vi "Evaluate Sum of Exponentials.vi"(8 "error in (no error)":errorcluster, 10 "Ramp":dbl[](array[numeric]), 11 "Exp Parameters Array":T1[](array[typedef])) -> (0 "error out":errorcluster, 3 "Plot":T2)   [LabVIEW 2021, in "Fits.lvlib"]
doc: "Evaluates a sum of T-periodic exponential terms whose parameters are provided as an array of components (<B>Exp Parameters Array</B>).\n\nThe <B>baseline</B> parameter needs to be provided with the first component. Additional baseline parameters are ignored.\n\nThis VI computes the exponential term as exp(-(t - t_0)[T}/tau) if parameter <B>sigma</B> is NaN.\n\nOtherwise, the exponential term is computed as exp(-(t - t_0)[T]/sigma^2).\n\nThe sum is evaluated at locations provided in the <B>Ramp</B> array."
uses:
  Fits.lvlib
  Graphs/XY Graph/XY Graph Plot Data.ctl
  1-Exp Parameters.ctl
  d5ce0044-42a5-46e1-a0a7-73280244e6ce.vi
  Graphs/XY Graph/XY Graph Add-Ons.lvlib
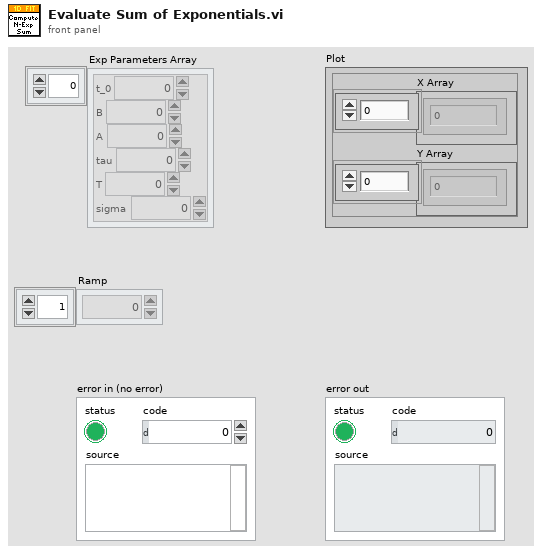
[diagram p1: front panel]
types:
  T1 = typedef "Fits.lvlib/1-Exp Parameters.ctl" = cluster{"t_0":dbl, "B":dbl, "A":dbl, "tau":dbl, "T":dbl, "sigma":dbl}
  T2 = typedef "XY Graph Add-Ons.lvlib/XY Graph Plot Data.ctl" = cluster{"X Array":dbl[], "Y Array":dbl[]}
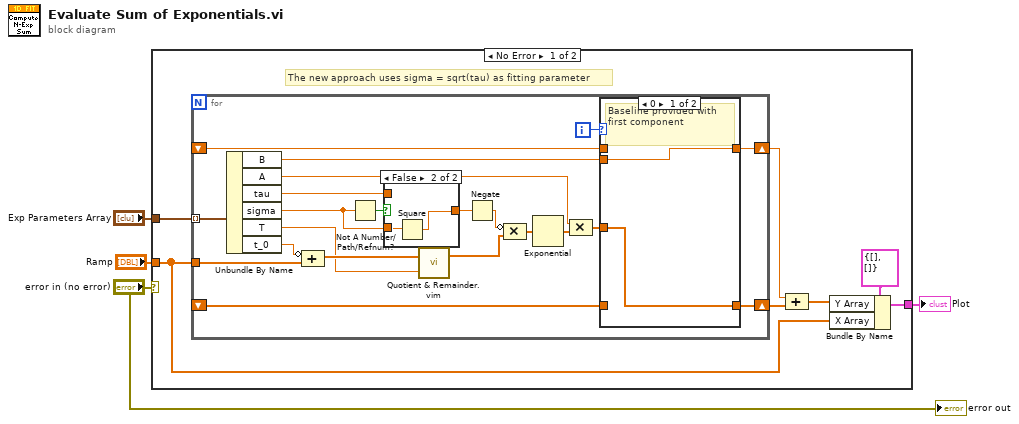
[diagram p0: block diagram]
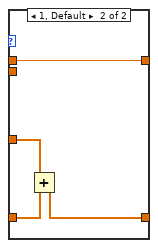
[diagram p3: hidden frame]
diagram:
  n1 = case shown="No Error" "error in (no error)" {
    tunnel: "Exp Parameters Array" -> [w11 _]
    tunnel: "Ramp" -> [w8 _]
    tunnel: [w9 _] -> w1
    frame No Error {
      # "The new approach uses sigma = sqrt(tau) as fitting parameter"
      n2 = for {
        tunnel: w11 -> [w32] mode=indexing
        tunnel: w8 -> [w31]
        shift-right: [w22] -> w10
        shift-left: _ -> [w21]
        shift-right: [w13] -> w5
        shift-left: _ -> [w12]
        i -> [w23]
        n3 = Unbundle By Name(w32) -> ("B"=w14:dbl, "A"=w25:dbl, "tau"=w16:dbl, "sigma"=w15:dbl, "T"=w19:dbl, "t_0"=w30:dbl)
        n4 = Compound Arithmetic op=unknown(invert w30, w31) -> (w29:dbl[])
        n5 = Not A Number/Path/Refnum?(number/path/refnum=w15) -> (NaN/Path/Refnum?=w18:bool)
        n6 = case shown="False" w18 {
          tunnel: [w33 w34] -> w17
          tunnel: w16 -> [w33 _]
          tunnel: w15 -> [_ w35]
          frame True {
          }
          frame False {
            n7 = Square(x=w35) -> (x^2=w34:dbl)
          }
        }
        n8 = call "Quotient & Remainder.vim"("y"=w19, "x"=w29) -> ("x - E(x/y)y"=w28:dbl[])  [unwired: 1 out]
        n9 = Negate(x=w17) -> (-x=w20:dbl)
        n10 = Compound Arithmetic op=MULTIPLY(invert w20, w28) -> (w27:dbl[])
        n11 = Exponential(1:w27) -> (0:w26:dbl[])
        n12 = Compound Arithmetic op=MULTIPLY(w25, w26) -> (w24:dbl[])
        n13 = case shown="0" w23 {
          tunnel: w24 -> [w37 w41]
          tunnel: [w37 w39] -> w22
          tunnel: w21 -> [_ w40]
          tunnel: w14 -> [w36 _]
          tunnel: [w36 w38] -> w13
          tunnel: w12 -> [_ w38]
          frame 0 {
            # "Baseline provided with first component"
          }
          frame 1, Default {
            n14 = Add(x=w41, y=w40) -> (x+y=w39:dbl[])
          }
        }
      }
      n15 = Compound Arithmetic op=ADD(w5, w10) -> (w6:dbl[])
      n16 = Bundle By Name(cluster=T2 {"X Array"=[], "Y Array"=[]} ("Plot"), "Y Array"=w6, "X Array"=w8) -> (w9:T2)
    }
    frame Error {
    }
  }
  "Plot" <- w1
  "error out" <- "error in (no error)"
